vi "WaitForBuffer.vi"(8 "error in (no error)":errorcluster, 11 "Server":path) -> (0 "error out":errorcluster, 2 "REPL":string)   [LabVIEW 2020]
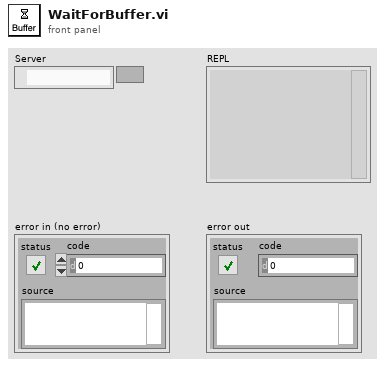
[diagram p1: front panel]
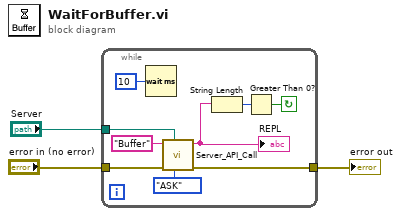
[diagram p0: block diagram]
diagram:
  n1 = while {
    tunnel: "error in (no error)" -> [w9]
    tunnel: "Server" -> [w10]
    tunnel: [w8] -> w2
    stop <- w12 continue-if-true
    n2 = Wait (ms)(milliseconds to wait=u32 10) -> ()  [unwired: 1 out]
    n3 = call "Server_API_Call.vi"("Server"=w10, "Direction"=enum16{"ASK", "TELL"}."ASK", "error in (no error)"=w9, "cmd"="Buffer") -> ("error out"=w8:errorcluster, "Read from Server"=w5:string)  [unwired: 5 in, 1 out]
    "REPL" <- w5
    n4 = String Length(string=w5) -> (length=w6:i32)
    n5 = Greater Than 0?(x=w6) -> (x > 0?=w12:bool)
  }
  "error out" <- w2
